vi "Project Points.vi"(6 "Camera Parameters":T6, 8 "error in (no error)":errorcluster, 10 "Pose":T3, 11 "Object Points":T1[](array[typedef])) -> (0 "error out":errorcluster, 3 "Image Points":T2[](array[typedef]))   [LabVIEW 2020, in "g_ar_toolkit.ar.lvlib"]
uses:
  g_ar_toolkit.ar.lvlib
  Camera Parameters.ctl
  Camera Matrix.ctl
  Camera Distortion Coefficients.ctl
  Pose.ctl
  rvec.ctl
  g_ar_toolkit.common/tvec.ctl
  g_ar_toolkit.common/Image Point (Float).ctl
  g_ar_toolkit.common/Object Point (Float).ctl
  g_ar_toolkit.common/g_ar_toolkit.common.lvlib
  bin/g_ar_toolkit.1.32.dll
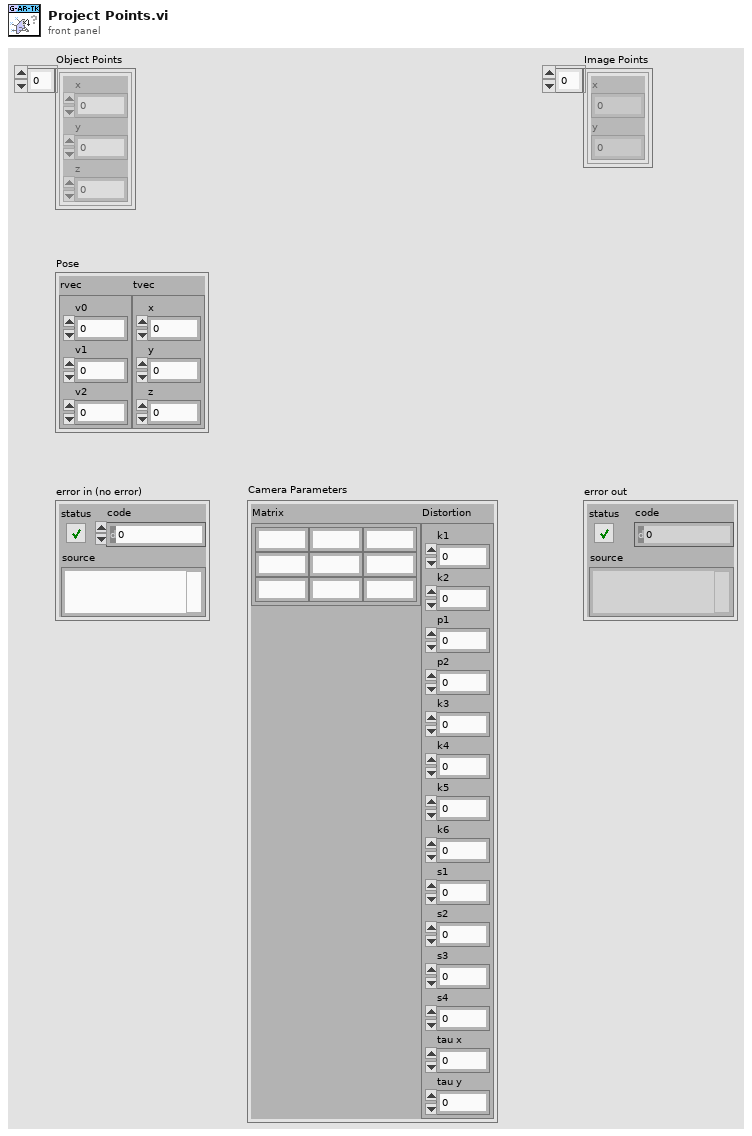
[diagram p1: front panel]
types:
  T1 = typedef "g_ar_toolkit.common.lvlib/Object Point (Float).ctl" = cluster{"x":dbl, "y":dbl, "z":dbl}
  T2 = typedef "g_ar_toolkit.common.lvlib/Image Point (Float).ctl" = cluster{"x":dbl, "y":dbl}
  T3 = typedef "g_ar_toolkit.ar.lvlib/Pose.ctl" = cluster{"rvec":T4, "tvec":T5}
  T4 = typedef "g_ar_toolkit.ar.lvlib/rvec.ctl" = cluster{"v0":dbl, "v1":dbl, "v2":dbl}
  T5 = typedef "g_ar_toolkit.ar.lvlib/tvec.ctl" = cluster{"x":dbl, "y":dbl, "z":dbl}
  T6 = typedef "g_ar_toolkit.ar.lvlib/Camera Parameters.ctl" = cluster{"Matrix":T7, "Distortion":T8}
  T7 = typedef "g_ar_toolkit.ar.lvlib/Camera Matrix.ctl" = cluster{"m 0,0":dbl, "m 0,1":dbl, "m 0,2":dbl, "m 1,0":dbl, "m 1,1":dbl, "m 1,2":dbl, "m 2,0":dbl, "m 2,1":dbl, "m 2,2":dbl}
  T8 = typedef "g_ar_toolkit.ar.lvlib/Camera Distortion Coefficients.ctl" = cluster{"k1":dbl, "k2":dbl, "p1":dbl, "p2":dbl, "k3":dbl, "k4":dbl, "k5":dbl, "k6":dbl, "s1":dbl, "s2":dbl, "s3":dbl, "s4":dbl, "tau x":dbl, "tau y":dbl}
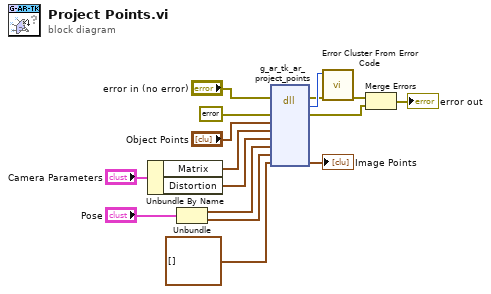
[diagram p0: block diagram]
diagram:
  n1 = Unbundle By Name("Camera Parameters") -> ("Matrix"=w10:T7, "Distortion"=w9:T8)
  n2 = Unbundle("Pose") -> ("rvec"=w3:T4, "tvec"=w2:T5)
  n3 = dll-call lib="C:/serenial/libraries/g-augmented-reality-toolkit/LabVIEW/bin/g_ar_toolkit.1.*.*" fn="g_ar_tk_ar_project_points" ("g_ar_toolkit.*.*:g_ar_tk_image_copy")(error in="error in (no error)", "error_cluster"=errorcluster {"status"=FALSE, "code"=0, "source"=""} ("error constant"), "object_points"="Object Points", "camera_matrix"=w10, "camera_distortion"=w9, "rvec"=w3, "tvec"=w2, "image_points"=T2[] [] ("Image Points")) -> (error out=w11:errorcluster, "MgErr"=w12:i32, "error_cluster"=w15:errorcluster, "image_points"=→"Image Points":T2[])  [unwired: 7 in, 1 out]
  n4 = call <vilib>:"Error Cluster From Error Code.vi"("error in (no error)"=w11, "error code (0)"=w12) -> ("error out"=w13:errorcluster)  [unwired: 7 in]
  n5 = Merge Errors(w13, w15) -> (→"error out":errorcluster)
